vi "SubTemplate_4x4x4_Create.vi"(8 "error in (no error)":errorcluster, 11 "reference in":refnum<class "SubTemplate_4x4x4.lvclass">) -> (0 "error out":errorcluster, 3 "reference out":refnum<class "SubTemplate_4x4x4.lvclass">)   [LabVIEW 2020, in "SubTemplate_4x4x4.lvclass"]
uses:
  <resource>/Framework/Providers/Open_GDS/ClassProviders/Provider_EndevoGOOP300/Templates/SubTemplate_4x4x4/SubTemplate_4x4x4.lvclass
  C:/Program Files (x86)/National Instruments/LabVIEW 2020/resource/Framework/Providers/Open_GDS/ClassProviders/Provider_EndevoGOOP300/Templates/BaseTemplate_4x4x4/BaseTemplate_4x4x4.lvclass
  <resource>/Framework/Providers/Open_GDS/ClassProviders/Provider_EndevoGOOP300/Templates/BaseTemplate_4x4x4/BaseTemplate_4x4x4.lvclass
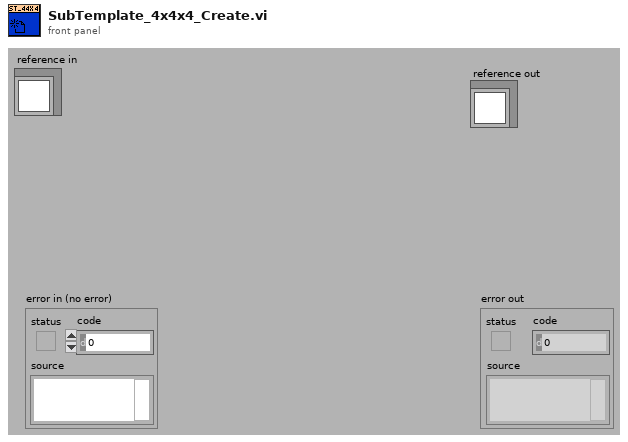
[diagram p1: front panel]
types:
  T1 = typedef "SubTemplate_4x4x4.lvclass/ObjectAttributes.ctl" = cluster{"Base class":T2}
  T2 = typedef "BaseTemplate_4x4x4.lvclass/ObjectAttributes.ctl" = cluster{"Attribute1":dbl}
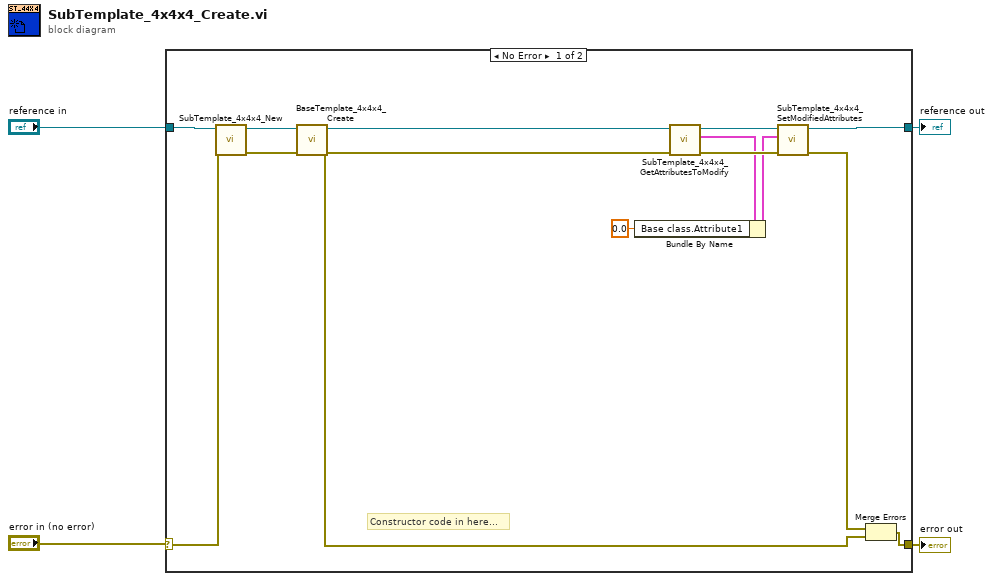
[diagram p0: block diagram]
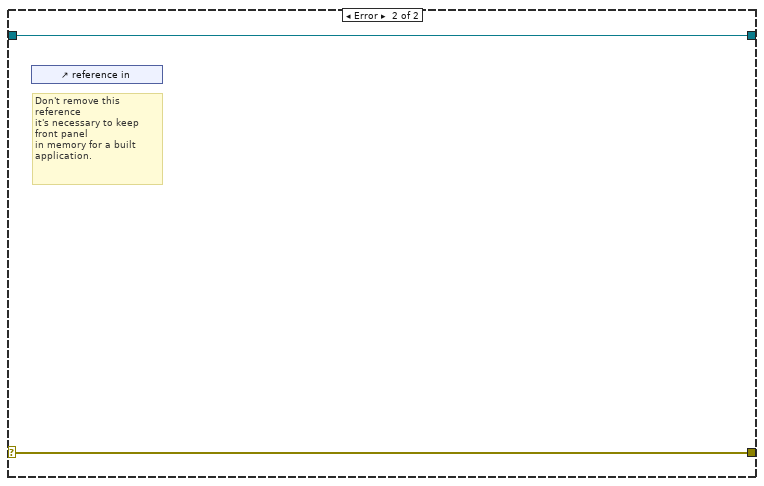
[diagram p2: hidden frame]
diagram:
  n1 = case shown="No Error" "error in (no error)" {
    selector: "error in (no error)" -> [w16 w20]
    tunnel: [w9 w20] -> w3
    tunnel: [w14 w19] -> w2
    tunnel: "reference in" -> [w6 w19]
    frame No Error {
      # "Constructor code in here..."
      n2 = call <resource>:"SubTemplate_4x4x4_New.vi"("error in (no error)"=w16, "reference in"=w6) -> ("error out"=w15:errorcluster, "reference out"=w11:refnum<class "SubTemplate_4x4x4.lvclass">)  [unwired: 6 in, 2 out]
      n3 = call <resource>:"BaseTemplate_4x4x4_Create.vi"("error in (no error)"=w15, "reference in"=w11) -> ("error out"=w7:errorcluster, "reference out"=w10:refnum<class "SubTemplate_4x4x4.lvclass">)  [unwired: 8 in]
      n4 = call <resource>:"SubTemplate_4x4x4_GetAttributesToModify.vi"("error in (no error)"=w7, "reference in"=w10) -> ("error out"=w17:errorcluster, "Attributes"=w13:T1, "reference out"=w18:refnum<class "SubTemplate_4x4x4.lvclass">)  [unwired: 6 in, 1 out]
      n5 = Bundle By Name(cluster=w13, "Base class.Attribute1"=0.0) -> (w12:T1)
      n6 = call <resource>:"SubTemplate_4x4x4_SetModifiedAttributes.vi"("error in (no error)"=w17, "Attributes"=w12, "reference in"=w18) -> ("error out"=w8:errorcluster, "reference out"=w14:refnum<class "SubTemplate_4x4x4.lvclass">)  [unwired: 7 in]
      n7 = Merge Errors(w8, w7) -> (w9:errorcluster)
    }
    frame Error {
      # "Don't remove this reference\nit's necessary to keep front panel\nin memory for a built application."
      n8 = control-ref of="reference in"() -> ()  [unwired: 1 out]
    }
  }
  "error out" <- w3
  "reference out" <- w2
